vi "UnFlattenXMLData.vi"() -> ()   [LabVIEW 2020]
uses:
  <vilib>/Utility/xml.llb/Read From XML File(array).vi
panel:
  out "String":string
  out "Temp Graph":cluster{"Xo":dbl, "delta X":dbl, dbl[]}(graph)={"Xo"=0.0, "delta X"=0.25, []}
  out "Min":dbl format="%0.2f"
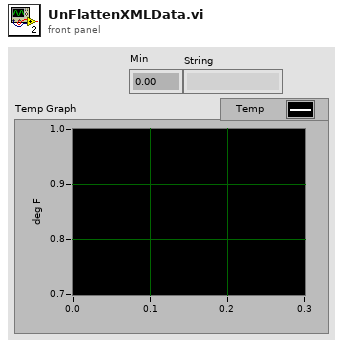
[diagram p1: front panel]
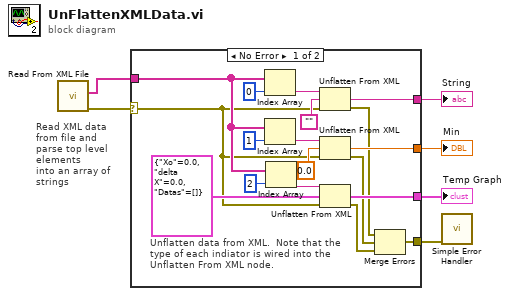
[diagram p0: block diagram]
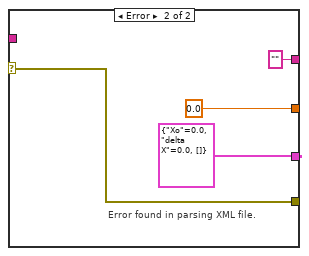
[diagram p2: hidden frame]
diagram:
  # "Read XML data from file and parse top level elements\ninto an array of strings"
  n1 = call-poly <vilib>:"Read From XML File.vi"() -> ("error out"=w4:errorcluster, "XML Elements"=w6:string[])  [unwired: 9 in, 1 out]
  n2 = case shown="No Error" w4 {
    selector: w4 -> [w9 w26]
    tunnel: w6 -> [w11 _]
    tunnel: [w18 0.0 ("Mean")] -> w3
    tunnel: [w17 cluster{"Xo":dbl, "delta X":dbl, dbl[]} {"Xo"=0.0, "delta X"=0.0, []} ("Temp Graph")] -> w5
    tunnel: [w16 w26] -> w2
    tunnel: [w8 ""] -> w1
    frame No Error {
      # "Unflatten data from XML.  Note that the \ntype of each indiator is wired into the\nUnflatten From XML node."
      n3 = Index Array(array=w11, index=0) -> (element=w13:string)
      n4 = Index Array(array=w11, index=1) -> (element=w21:string)
      n5 = Index Array(array=w11, index=2) -> (element=w19:string)
      n6 = Unflatten From XML(xml string=w13, type="", error in (no error)=w9) -> (value=w8:string, error out=w7:errorcluster)
      n7 = Unflatten From XML(xml string=w21, type=0.0 ("Mean"), error in (no error)=w9) -> (value=w18:dbl, error out=w15:errorcluster)
      n8 = Unflatten From XML(xml string=w19, type=cluster{"Xo":dbl, "delta X":dbl, "Datas":dbl[]} {"Xo"=0.0, "delta X"=0.0, "Datas"=[]} ("Temp Graph"), error in (no error)=w9) -> (value=w17:cluster{"Xo":dbl, "delta X":dbl, "Datas":dbl[]}, error out=w14:errorcluster)
      n9 = Merge Errors(w7, w15, w14) -> (w16:errorcluster)
    }
    frame Error {
      # "Error found in parsing XML file."
    }
  }
  "Min" <- w3
  "Temp Graph" <- w5
  "String" <- w1
  n10 = call <vilib>:"Simple Error Handler.vi"("error in (no error)"=w2) -> ()  [unwired: 4 in, 5 out]
